vi "Text File Numeric Searcher.vi"(9 "String":string, 11 "file (use dialog)":path) -> (1 "Numeric Array":dbl[](array[numeric]), 3 "String Array":string[](array[string]))   [LabVIEW 2014]
panel:
  # "Outputs"
  # "Inputs"
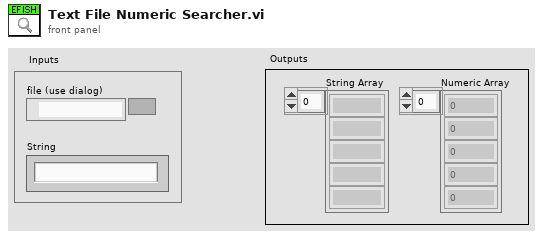
[diagram p1: front panel]
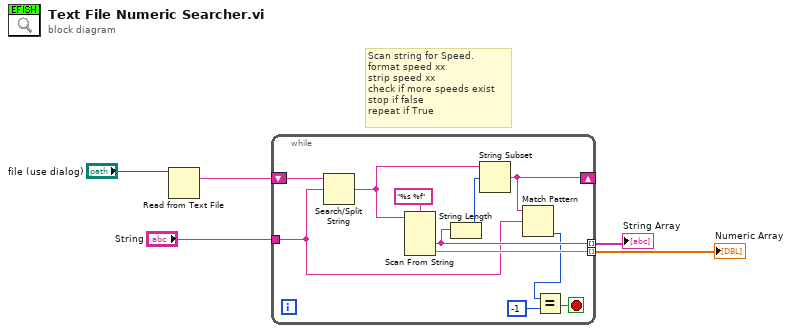
[diagram p0: block diagram]
diagram:
  # "Scan string for Speed.\nformat speed xx\nstrip speed xx\ncheck if more speeds exist\nstop if false\nrepeat if True"
  n1 = Read from Text File(file (use dialog)="file (use dialog)") -> (text=w4:string)  [unwired: 3 in, 3 out]
  n2 = while {
    tunnel: [w12] -> w5 mode=indexing
    shift-right: [w7] -> _
    shift-left: w4 -> [w15]
    tunnel: [w13] -> w3 mode=indexing
    tunnel: "String" -> [w6]
    stop <- w10 stop-if-true
    n3 = Search/Split String(string=w15, search string/char (-)=w6) -> (match + rest of string=w9:string)  [unwired: 1 in, 2 out]
    n4 = Scan From String(format string="%s %f", input string=w9) -> (output 1=w12:string, output 2=w13:dbl)  [unwired: 4 in, 3 out]
    n5 = String Length(string=w12) -> (length=w11:i32)
    n6 = String Subset(string=w9, offset (0)=w11) -> (substring=w7:string)  [unwired: 1 in]
    n7 = Match Pattern(string=w7, regular expression=w6) -> (offset past match=w8:i32)  [unwired: 1 in, 3 out]
    n8 = Equal?(x=w8, y=-1) -> (x = y?=w10:bool)
  }
  "String Array" <- w5
  "Numeric Array" <- w3
